vi "Gaussian Monopulse.vi"(7 "center frequency (Hz)":dbl=0.1, 8 "delta t (s)":dbl=0.1, 9 "delay (s)":dbl, 10 "amplitude":dbl=1.0, 11 "samples":i32=128) -> (0 "error":i32, 3 "Gaussian Monopulse":dbl[](array[numeric]))   [LabVIEW 2013, in "NI_AALBase.lvlib"]
doc: "Generates an array that contains a Gaussian monopulse."
uses:
  NI_AALBase.lvlib
panel:
  # "Gaussian Monopulse"
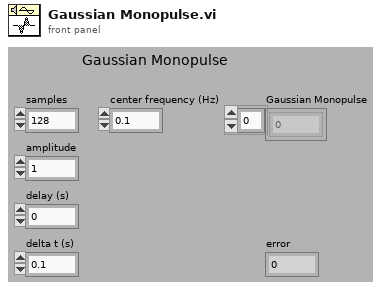
[diagram p1: front panel]
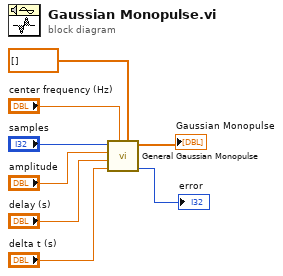
[diagram p0: block diagram]
diagram:
  n1 = call "General Gaussian Monopulse.vi"("X"=dbl[] [], "center frequency"="center frequency (Hz)", "delta t"="delta t (s)", "delay"="delay (s)", "amplitude"="amplitude", "samples"="samples") -> ("error"=→"error":i32, "Gaussian Monopulse"=→"Gaussian Monopulse":dbl[])  [unwired: 4 in]
